vi "GlobalUI.vi"() -> ()   [LabVIEW 2012]
uses:
  typedefs/Scan Parameters.ctl
  typedefs/HWsettings.ctl
  typedefs/Stage Parameters.ctl
  typedefs/ScanMode.ctl
  classes/MCCPMT.lvclass
  typedefs/Scan Type.ctl
  typedefs/Move Type.ctl
  typedefs/MicroscopeEvent.ctl
  typedefs/Filenaming.ctl
panel:
  in  "Reading threshold defaults":dbl[](array[numeric])=[0.0, 0.0, 0.0]
  in  "Reading thresholds":dbl[](array[numeric])=[0.0, 0.0, 0.0]
  in  "Filenaming Mode":T1
  out "Microscope Events":refnum<queue>
  in  "configuration file":path=path "C:/Users/Trent/Dropbox/Shared/Jeremy/microscoper 2012/ConfigFiles/Jeremy.ini"
  out "SW Initializing":bool
  out "Image Initialized":bool
  out "Number of scans to average":u32=1
  in  "Stage":refnum<k7>(container)
  in  "Stage Serial Number":i32=94839332
  out "# elements in queue":i32
  out "Rotation Acquire Ready?":bool
  in  "Move Type":T2=enum."Continuous"
  in  "Scan Type":T3=enum."Point"
  out "Integration Time (ms)":u32=83
  in  "MakeAcquireButtonFalse":bool
  out "acquiring":bool
  out "MCCPMT":refnum<class "MCCPMT.lvclass">
  out "error out":errorcluster
  in  "detector startup delay (ms)":u32=1000
  out "Stage Position (mm)":dbl=77.27864837646484
  out "Samples Averaged":dbl=82.0
  out "Samples Per Line":dbl=6150.0
  out "Flyback samples":dbl=25.0
  in  "Zoom":dbl=4.0
  in  "Target position mm":dbl=82.4884 step=0.025 format="%_6g"
  in  "Target position mm 2":dbl=78.45775 step=0.025 format="%_6g"
  in  "Target position mm 3":dbl=77.0 step=0.025 format="%_6g"
  in  "Velocity mm/s":sgl=5.0 min=0.01 max=10 step=0.1
  out "PMT3 on":bool
  out "PMT2 on":bool
  out "PMT1 on":bool
  in  "Get Stage Position":bool
  in  "Acquire":bool
  out "Cursor Y (V)":dbl=-0.8695652173913044
  out "Cursor X (V)":dbl=1.2532299741602064
  out "Detector Timebase divisor":i32=13
  out "Actual write rate":dbl=18761.72607879925
  out "Expected write rate":dbl=18761.72607879925
  out "Actual read rate":dbl=1538461.5384615385
  out "must be an integer":dbl=82.0
  out "Galvo Timebase divisor":i32=1066
  out "Intensity x label":string="Time Elapsed (s)"
  in  "Save Path":path=path "C:/Users/Trent/Documents/Jeremy"
  out "Intensity vs Stage Position (mm)":cluster{dbl[], dbl[]}[](array[cluster])=[{[0.0, 1.3910799026489258, 1.5990915298461914, 1.8071036338806152, 2.015115261077881, 2.2071261405944824, 2.4151382446289062, 2.62214994430542, 2.8301620483398438, 3.0221729278564453, 3.230185031890869, 3.4381966590881348, 3.6462087631225586, 3.83821964263916, 4.046231746673584, 4.253243446350098, 4.4612555503845215, 4.653266429901123, 4.861278057098389, 5.0692901611328125, 5.277301788330078, 5.469313144683838, 5.6773247718811035, 5.884336948394775, 6.092348575592041, 6.284359455108643, 6.492371559143066, 6.700383186340332, 6.908395290374756, 7.100406169891357, 7.308418273925781], [0.000122149923780488, 0.00012203887195121974, 0.00012211684451219482, 0.00012205836509146326, 0.00012210857469512214, 0.00012208849085365822, 0.0001219922065548779, 0.0001221192073170731, 0.00012216291920731678, 0.00012211270960365853, 0.00012210562118902425, 0.00012214874237804877, 0.00012212511432926825, 0.00012211625381097538, 0.00012212097942073178, 0.00012209912347560983, 0.00012205127667682942, 0.00012203414634146332, 0.00012206781631097554, 0.00012200815548780514, 0.00012220367759146314, 0.00012232418064024334, 0.00012240865091463348, 0.0001225149771341453, 0.0001225834984756086, 0.00012261126143292585, 0.00012276897865853544, 0.00012285640243902307, 0.0001228445884146327, 0.00012293732850609658]}, {[0.0, 1.3910799026489258, 1.5990915298461914, 1.8071036338806152, 2.015115261077881, 2.2071261405944824, 2.4151382446289062, 2.62214994430542, 2.8301620483398438, 3.0221729278564453, 3.230185031890869, 3.4381966590881348, 3.6462087631225586, 3.83821964263916, 4.046231746673584, 4.253243446350098, 4.4612555503845215, 4.653266429901123, 4.861278057098389, 5.0692901611328125, 5.277301788330078, 5.469313144683838, 5.6773247718811035, 5.884336948394775, 6.092348575592041, 6.284359455108643, 6.492371559143066, 6.700383186340332, 6.908395290374756, 7.100406169891357, 7.308418273925781], [0.00013135659298780475, 0.00013157338033536578, 0.00013012616234756093, 0.00013111440548780457, 0.00013301646341463397, 0.0001317883955792678, 0.000130992721036585, 0.0001326821265243906, 0.0001315072217987802, 0.0001293440739329267, 0.00013089761814024363, 0.00013007063643292666, 0.00012964237804878018, 0.00013161945503048738, 0.00012965419207317062, 0.00012840544969512196, 0.00012788208841463418, 0.00012783955792682928, 0.00012841371951219504, 0.00012860569740853655, 0.00012810419207317093, 0.00012816326219512175, 0.00012866535823170694, 0.00012888568978658576, 0.0001280764291158539, 0.00012789980945121965, 0.0001284456173780486, 0.00013150131478658524, 0.00012812073170731704, 0.00012772318978658532]}, {[0.0, 1.3910799026489258, 1.5990915298461914, 1.8071036338806152, 2.015115261077881, 2.2071261405944824, 2.4151382446289062, 2.62214994430542, 2.8301620483398438, 3.0221729278564453, 3.230185031890869, 3.4381966590881348, 3.6462087631225586, 3.83821964263916, 4.046231746673584, 4.253243446350098, 4.4612555503845215, 4.653266429901123, 4.861278057098389, 5.0692901611328125, 5.277301788330078, 5.469313144683838, 5.6773247718811035, 5.884336948394775, 6.092348575592041, 6.284359455108643, 6.492371559143066, 6.700383186340332, 6.908395290374756, 7.100406169891357, 7.308418273925781], [0.0015331301638719503, 0.0015423486471036582, 0.0015469194931402445, 0.0015383738185975615, 0.001518318330792681, 0.0015139979420731706, 0.0015096173018292658, 0.00150134630335366, 0.0014566284489329268, 0.0014108739138719547, 0.0014768062118902425, 0.0014940812690548806, 0.0015152945312499973, 0.0015447988757621935, 0.0014241475609756108, 0.0014025462080792695, 0.0013903263719512208, 0.001438070388719513, 0.0014299364329268304, 0.0014168329077743902, 0.0014394319550304904, 0.001461583841463416, 0.0014690036394817024, 0.0014612311928353645, 0.0014412194169207292, 0.0014495364900914622, 0.001426015948932925, 0.0014652012957317051, 0.0014510108803353662, 0.0014339579268292664]}]
  out "Image intensities":dbl[](array[numeric])
  out "Images":dbl[][][](array[numeric])
  in  "Maximum frame diff":i32=1
  in  "Use Image Controls Min Max values for tiff":bool=TRUE
  in  "Autosave":bool
  in  "show flyback data":bool
  in  "disable averaging":bool
  in  "Sample Description":string="AXN static 25d"
  in  "Stokes Power (mW)":string="200"
  in  "Pump Power (mW)":string="5"
  in  "PMT3":dbl(slide)=0.7 min=0.0 max=1.0 step=0.01 scale=0.0..1.0
  in  "PMT2":dbl(slide)=0.7 min=0.0 max=1.0 step=0.01 scale=0.0..1.0
  in  "PMT1":dbl(slide)=0.6 min=0.0 max=1.0 step=0.01 scale=0.0..1.0 scale format="%#_1g"
  out "Grabbed all required frames? (image processor)":bool
  out "image  maximums":dbl[](array[numeric])=[250.0, 250.0, 500.0]
  out "image  minimums":dbl[](array[numeric])=[0.0, 0.0, 283.1435785060976]
  in  "status":string[](array[string])=["Initializing", "Setting parameters", "Initializing", "Setting parameters", "Initializing", "Setting parameters", "closing image data", "Setting acquire button to false", "Setting acquire button to false", "closing image data", "stopping acquisition", "Acquire sequence set", "closing image data", "post acquire", "acquiring", "initializing image data", "closing image data", "pre-acquiring", "initializing galvos and detectors", "preparing stage", "initializing image data", "closing image data", "Setting parameters", "Acquire sequence set", "Initializing", "Setting parameters", "Setting parameters", "Setting parameters", "initializing image data", "closing image data", "post acquire", "acquiring", "pre-acquiring", "initializing galvos and detectors", "preparing stage", "Setting parameters", "preparing to acquire", "Wait for event", "Setting acquire button to false", "stopping acquisition", "preparing to acquire", "Wait for event", "post acquire", "initializing image data", "acquiring", "Wait for event", "pre-acquiring", "initializing galvos and detectors", "enabling acquire buttons", "Setting parameters", "post acquire", "initializing image data", "acquiring", "pre-acquiring", "initializing galvos and detectors", "enabling acquire buttons", "Setting parameters", "Wait for event", "post acquire", "initializing image data", "acquiring", "pre-acquiring", "initializing galvos and detectors", "enabling acquire buttons", "Setting parameters", "Wait for event", "post acquire", "initializing image data", "acquiring", "Wait for event", "pre-acquiring", "initializing galvos and detectors", "enabling acquire buttons", "Setting parameters", "post acquire", "initializing image data", "acquiring", "Wait for event", "pre-acquiring", "initializing galvos and detectors", "enabling acquire buttons", "Setting parameters", "post acquire", "initializing image data", "acquiring", "pre-acquiring", "initializing galvos and detectors", "enabling acquire buttons", "Setting parameters", "Wait for event", "post acquire", "initializing image data", "acquiring", "pre-acquiring", "initializing galvos and detectors", "enabling acquire buttons", "Setting parameters", "Wait for event", "post acquire", "initializing image data", "acquiring", "Wait for event", "pre-acquiring", "initializing galvos and detectors", "enabling acquire buttons", "Setting parameters", "post acquire", "initializing image data", "acquiring", "Wait for event", "pre-acquiring", "initializing galvos and detectors", "enabling acquire buttons", "Setting parameters", "Wait for event", "Wait for event", "post acquire", "initializing image data", "acquiring", "pre-acquiring", "initializing galvos and detectors", "enabling acquire buttons", "Setting parameters", "Wait for event", "post acquire", "initializing image data", "acquiring", "pre-acquiring", "initializing galvos and detectors", "preparing stage", "Setting parameters", "preparing to acquire", "Wait for event", "moving stage to 3rd option", "Setting parameters", "Initializing", "Setting parameters", "Initializing", "Setting parameters", "Bumming", "restoring to default state", "Bumming", "stopping acquisition", "Bumming", "preparing to acquire", "closing image data", "post acquire", "processing image", "initializing image data", "processing image", "initializing image data", "acquiring", "pre-acquiring", "initializing galvos and detectors", "preparing stage", "getting parameters", "preparing to acquire", "Bumming", "moving stage to 3rd option", "getting parameters", "Bumming", "stopping acquisition", "restoring to default state", "post acquire", "processing image", "initializing image data", "processing image", "initializing image data", "closing image data", "acquiring", "pre-acquiring", "initializing galvos and detectors", "preparing stage", "getting parameters", "preparing to acquire", "Bumming", "restoring to default state", "Bumming", "stopping acquisition", "Bumming", "preparing to acquire", "post acquire", "processing image", "initializing image data", "processing image", "initializing image data", "acquiring", "pre-acquiring", "initializing galvos and detectors", "preparing stage", "getting parameters", "preparing to acquire", "Bumming", "moving stage to 3rd option", "getting parameters", "Bumming", "stopping acquisition", "restoring to default state", "post acquire", "processing image", "initializing image data", "processing image", "initializing image data", "closing image data", "acquiring", "pre-acquiring", "initializing galvos and detectors", "preparing stage", "getting parameters", "preparing to acquire", "Bumming", "restoring to default state", "Bumming", "stopping acquisition", "Bumming", "preparing to acquire", "post acquire", "processing image", "initializing image data", "processing image", "initializing image data", "acquiring", "pre-acquiring", "initializing galvos and detectors", "preparing stage", "getting parameters", "preparing to acquire", "Bumming", "moving stage to 3rd option", "getting parameters", "Bumming", "stopping acquisition", "restoring to default state", "post acquire", "processing image", "initializing image data", "processing image", "initializing image data", "acquiring", "pre-acquiring", "initializing galvos and detectors", "preparing stage", "getting parameters", "preparing to acquire", "Bumming", "restoring to default state", "Bumming", "stopping acquisition", "Bumming", "preparing to acquire", "closing image data", "post acquire", "reinitializing image data parameters", "closing image data", "acquiring", "pre-acquiring", "initializing galvos and detectors", "enabling acquire buttons", "getting parameters", "moving stage to 3rd option", "getting parameters", "Bumming", "post acquire", "processing image", "initializing image data", "processing image", "initializing image data", "acquiring", "pre-acquiring", "initializing galvos and detectors", "preparing stage", "getting parameters", "preparing to acquire", "Bumming", "stopping acquisition", "restoring to default state", "post acquire", "processing image", "initializing image data", "processing image", "initializing image data", "acquiring", "pre-acquiring", "initializing galvos and detectors", "preparing stage", "getting parameters", "preparing to acquire", "Bumming", "restoring to default state", "Bumming", "stopping acquisition", "Bumming", "preparing to acquire", "closing image data", "post acquire", "processing image", "initializing image data", "acquiring", "pre-acquiring", "initializing galvos and detectors", "preparing stage", "getting parameters", "preparing to acquire", "Bumming", "restoring to default state", "Bumming", "stopping acquisition", "Bumming", "preparing to acquire", "closing image data", "post acquire", "processing image", "initializing image data", "processing image", "initializing image data", "processing image", "initializing image data", "acquiring", "pre-acquiring", "initializing galvos and detectors", "preparing stage", "getting parameters", "preparing to acquire", "Bumming", "getting parameters", "Bumming", "restoring to default state", "Bumming", "stopping acquisition", "Bumming", "preparing to acquire", "closing image data", "post acquire", "processing image", "initializing image data", "closing image data", "acquiring", "pre-acquiring", "initializing galvos and detectors", "enabling acquire buttons", "getting parameters", "Bumming", "post acquire", "processing image", "initializing image data", "closing image data", "acquiring", "pre-acquiring", "initializing galvos and detectors", "preparing stage", "getting parameters", "preparing to acquire", "Bumming", "restoring to default state", "Bumming", "stopping acquisition", "Bumming", "preparing to acquire", "post acquire", "processing image", "initializing image data", "processing image", "initializing image data", "acquiring", "pre-acquiring", "initializing galvos and detectors", "preparing stage", "getting parameters", "preparing to acquire", "Bumming", "moving stage to 3rd option", "getting parameters", "Bumming", "restoring to default state", "Bumming", "stopping acquisition", "Bumming", "stopping acquisition", "restoring to default state", "preparing to acquire", "post acquire", "processing image", "initializing image data", "processing image", "initializing image data", "acquiring", "pre-acquiring", "initializing galvos and detectors", "preparing stage", "getting parameters", "preparing to acquire", "Bumming", "restoring to default state", "Bumming", "stopping acquisition", "Bumming", "preparing to acquire", "closing image data", "post acquire", "reinitializing image data parameters", "acquiring", "pre-acquiring", "initializing galvos and detectors", "enabling acquire buttons", "getting parameters", "Bumming", "closing image data", "post acquire", "reinitializing image data parameters", "acquiring", "pre-acquiring", "initializing galvos and detectors", "enabling acquire buttons", "getting parameters", "Bumming", "closing image data", "post acquire", "reinitializing image data parameters", "closing image data", "acquiring", "pre-acquiring", "initializing galvos and detectors", "enabling acquire buttons", "getting parameters", "Bumming", "post acquire", "processing image", "initializing image data", "closing image data", "acquiring", "pre-acquiring", "initializing galvos and detectors", "enabling acquire buttons", "getting parameters", "Bumming", "post acquire", "reinitializing image data parameters", "acquiring", "pre-acquiring", "initializing galvos and detectors", "enabling acquire buttons", "getting parameters", "moving stage to 3rd option", "getting parameters", "Bumming", "closing image data", "post acquire", "processing image", "initializing image data", "closing image data", "acquiring", "pre-acquiring", "initializing galvos and detectors", "enabling acquire buttons", "getting parameters", "Bumming", "post acquire", "reinitializing image data parameters", "acquiring", "pre-acquiring", "initializing galvos and detectors", "enabling acquire buttons", "getting parameters", "moving stage to 3rd option", "getting parameters", "Bumming", "closing image data", "post acquire", "reinitializing image data parameters", "acquiring", "pre-acquiring", "initializing galvos and detectors", "enabling acquire buttons", "getting parameters", "moving stage to 3rd option", "getting parameters", "Bumming", "closing image data", "post acquire", "processing image", "initializing image data", "acquiring", "pre-acquiring", "initializing galvos and detectors", "preparing stage", "getting parameters", "preparing to acquire", "Bumming", "restoring to default state", "Bumming", "stopping acquisition", "Bumming", "preparing to acquire", "closing image data", "post acquire", "reinitializing image data parameters", "closing image data", "acquiring", "pre-acquiring", "initializing galvos and detectors", "enabling acquire buttons", "getting parameters", "moving stage to 3rd option", "getting parameters", "Bumming", "post acquire", "reinitializing image data parameters", "acquiring", "pre-acquiring", "initializing galvos and detectors", "enabling acquire buttons", "getting parameters", "moving stage to 3rd option", "getting parameters", "Bumming", "closing image data", "post acquire", "reinitializing image data parameters", "acquiring", "pre-acquiring", "initializing galvos and detectors", "enabling acquire buttons", "getting parameters", "moving stage to 3rd option", "getting parameters", "Bumming", "closing image data", "post acquire", "reinitializing image data parameters", "acquiring", "pre-acquiring", "initializing galvos and detectors", "enabling acquire buttons", "getting parameters", "moving stage to 3rd option", "getting parameters", "Bumming", "closing image data", "post acquire", "reinitializing image data parameters", "acquiring", "pre-acquiring", "initializing galvos and detectors", "enabling acquire buttons", "getting parameters", "moving stage to 3rd option", "getting parameters", "Bumming", "Bumming", "closing image data", "post acquire", "processing image", "initializing image data", "acquiring", "pre-acquiring", "initializing galvos and detectors", "preparing stage", "getting parameters", "preparing to acquire", "Bumming", "restoring to default state", "Bumming", "stopping acquisition", "Bumming", "preparing to acquire", "closing image data", "post acquire", "reinitializing image data parameters", "acquiring", "pre-acquiring", "initializing galvos and detectors", "enabling acquire buttons", "getting parameters", "moving stage to 3rd option", "getting parameters", "Bumming", "closing image data", "post acquire", "reinitializing image data parameters", "closing image data", "acquiring", "pre-acquiring", "initializing galvos and detectors", "enabling acquire buttons", "getting parameters", "moving stage to 3rd option", "getting parameters", "Bumming", "post acquire", "reinitializing image data parameters", "closing image data", "acquiring", "pre-acquiring", "initializing galvos and detectors", "enabling acquire buttons", "getting parameters", "moving stage to 3rd option", "getting parameters", "Bumming", "post acquire", "reinitializing image data parameters", "acquiring", "pre-acquiring", "initializing galvos and detectors", "enabling acquire buttons", "getting parameters", "moving stage to 3rd option", "getting parameters", "Bumming", "closing image data", "post acquire", "processing image", "initializing image data", "closing image data", "acquiring", "pre-acquiring", "initializing galvos and detectors", "preparing stage", "getting parameters", "preparing to acquire", "Bumming", "restoring to default state", "Bumming", "stopping acquisition", "Bumming", "preparing to acquire", "Bumming", "Bumming", "Bumming", "post acquire", "reinitializing image data parameters", "acquiring", "pre-acquiring", "initializing galvos and detectors", "enabling acquire buttons", "getting parameters", "moving stage to 2nd option", "getting parameters", "Bumming", "closing image data", "post acquire", "reinitializing image data parameters", "acquiring", "pre-acquiring", "initializing galvos and detectors", "enabling acquire buttons", "getting parameters", "moving stage to 1st option", "getting parameters", "Bumming", "closing image data", "post acquire", "processing image", "initializing image data", "closing image data", "acquiring", "pre-acquiring", "initializing galvos and detectors", "enabling acquire buttons", "getting parameters", "Bumming", "post acquire", "processing image", "initializing image data", "acquiring", "pre-acquiring", "initializing galvos and detectors", "enabling acquire buttons", "getting parameters", "Bumming", "closing image data", "post acquire", "processing image", "initializing image data", "acquiring", "pre-acquiring", "initializing galvos and detectors", "enabling acquire buttons", "getting parameters", "Bumming", "closing image data", "post acquire", "reinitializing image data parameters", "acquiring", "pre-acquiring", "initializing galvos and detectors", "enabling acquire buttons", "getting parameters", "moving stage to 3rd option", "getting parameters", "Bumming", "closing image data", "post acquire", "reinitializing image data parameters", "acquiring", "pre-acquiring", "initializing galvos and detectors", "enabling acquire buttons", "getting parameters", "moving stage to 3rd option", "getting parameters", "Bumming", "closing image data", "post acquire", "reinitializing image data parameters", "acquiring", "pre-acquiring", "initializing galvos and detectors", "enabling acquire buttons", "getting parameters", "moving stage to 3rd option", "getting parameters", "Bumming", "closing image data", "post acquire", "reinitializing image data parameters", "acquiring", "pre-acquiring", "initializing galvos and detectors", "enabling acquire buttons", "getting parameters", "moving stage to 3rd option", "getting parameters", "Bumming", "closing image data", "post acquire", "processing image", "initializing image data", "acquiring", "pre-acquiring", "initializing galvos and detectors", "preparing stage", "getting parameters", "preparing to acquire", "Bumming", "restoring to default state", "Bumming", "stopping acquisition", "Bumming", "preparing to acquire", "closing image data", "post acquire", "processing image", "initializing image data", "acquiring", "pre-acquiring", "initializing galvos and detectors", "enabling acquire buttons", "getting parameters", "Bumming", "closing image data", "post acquire", "processing image", "initializing image data", "acquiring", "pre-acquiring", "initializing galvos and detectors", "enabling acquire buttons", "getting parameters", "Bumming", "closing image data", "post acquire", "processing image", "initializing image data", "acquiring", "pre-acquiring", "initializing galvos and detectors", "enabling acquire buttons", "getting parameters", "Bumming", "closing image data", "post acquire", "processing image", "initializing image data", "acquiring", "pre-acquiring", "initializing galvos and detectors", "enabling acquire buttons", "getting parameters", "Bumming", "closing image data", "post acquire", "processing image", "initializing image data", "acquiring", "pre-acquiring", "initializing galvos and detectors", "preparing stage", "getting parameters", "preparing to acquire", "Bumming", "restoring to default state", "Bumming", "stopping acquisition", "Bumming", "preparing to acquire", "closing image data", "post acquire", "processing image", "initializing image data", "acquiring", "pre-acquiring", "initializing galvos and detectors", "preparing stage", "getting parameters", "preparing to acquire", "Bumming", "restoring to default state", "Bumming", "stopping acquisition", "Bumming", "preparing to acquire", "closing image data", "post acquire", "processing image", "initializing image data", "processing image", "initializing image data", "acquiring", "pre-acquiring", "initializing galvos and detectors", "preparing stage", "getting parameters", "preparing to acquire", "Bumming", "Bumming", "moving stage to 3rd option", "getting parameters", "Bumming", "Bumming", "Bumming", "Bumming", "Bumming", "Bumming", "Bumming", "Bumming", "Bumming", "Bumming", "stopping acquisition", "restoring to default state", "post acquire", "processing image", "initializing image data", "processing image", "initializing image data", "acquiring", "pre-acquiring", "initializing galvos and detectors", "preparing stage", "getting parameters", "preparing to acquire", "Bumming", "restoring to default state", "Bumming", "stopping acquisition", "Bumming", "stopping acquisition", "restoring to default state", "preparing to acquire", "post acquire", "processing image", "initializing image data", "processing image", "initializing image data", "acquiring", "pre-acquiring", "initializing galvos and detectors", "preparing stage", "getting parameters", "preparing to acquire", "Bumming", "restoring to default state", "Bumming", "stopping acquisition", "Bumming", "preparing to acquire", "closing image data", "post acquire", "processing image", "initializing image data", "acquiring", "pre-acquiring", "initializing galvos and detectors", "preparing stage", "getting parameters", "preparing to acquire", "Bumming", "Bumming", "Getting ready for you", "getting parameters", "starting up!"]
  in  "Stage Acquire Parameters":T4={"Scan Mode"=enum."None", "Start position mm"=79.5, "End position mm"=83.0, "Velocity um/sec (continuous)"=100.0, "Step size microns (discrete)"=100.0, "Frames to grab (grab)"=1} {"Frames to grab (grab)" min=1 step=1; "Velocity um/sec (continuous)" min=0.1 max=10000.0 step=1.0 format="%.1f"; "End position mm" min=0.0 max=220.0 step=0.1 format="%_6g"; "Start position mm" min=0.0 max=220.0 step=0.1 format="%_6g"; "Step size microns (discrete)" min=0.1 max=1000.0 step=1.0 format="%.1f"}
  in  "Hardware Settings":T6={"Galvo Channels"="Dev1/ao0:1", "Detector Channels"="Dev1/ai0:2", "Galvo Trigger"="/Dev1/ai/StartTrigger", "Shutter Lines"=["Dev1/port0/line7"], "Max Acquisition Rate"=5000000.0, "Recommended Acquisition Rate"=5000000.0, "Galvo Write Rate"=2500000.0, "Max Timebase Frequency (Hz)"=20000000.0, "MCC Shutter Lines"=["Dev0/AuxPort/Do1", "Dev0/AuxPort/Do2"], "Detector Task"="", "Shutter Tasks"=[], "Galvo Task"="", "Digital Image Multiplier"=[100.0, 100.0, 100.0]} {"Max Acquisition Rate" min=0.0 max=5000000.0 step=100000.0}
  in  "Scan Parameters":T7={"x pixels"=50, "x voltage min"=-7.0, "x voltage max"=9.0, "y voltage min"=-8.75, "y voltage max"=7.25, "fill frac"=0.5, "Zoom"=4.0, "BiDi"=FALSE, "scan rate (ms/line)"=4.0} {"fill frac" min=0.0 step=0.05 format="%.2f"; "y voltage max" format="%0.2p"; "y voltage min" format="%.2f"; "x voltage max" format="%0.2p"; "x voltage min" format="%0.2p"}
  out "Images Displayed":i32
  out "Images Acquired":i32
  # "Stage Variables"
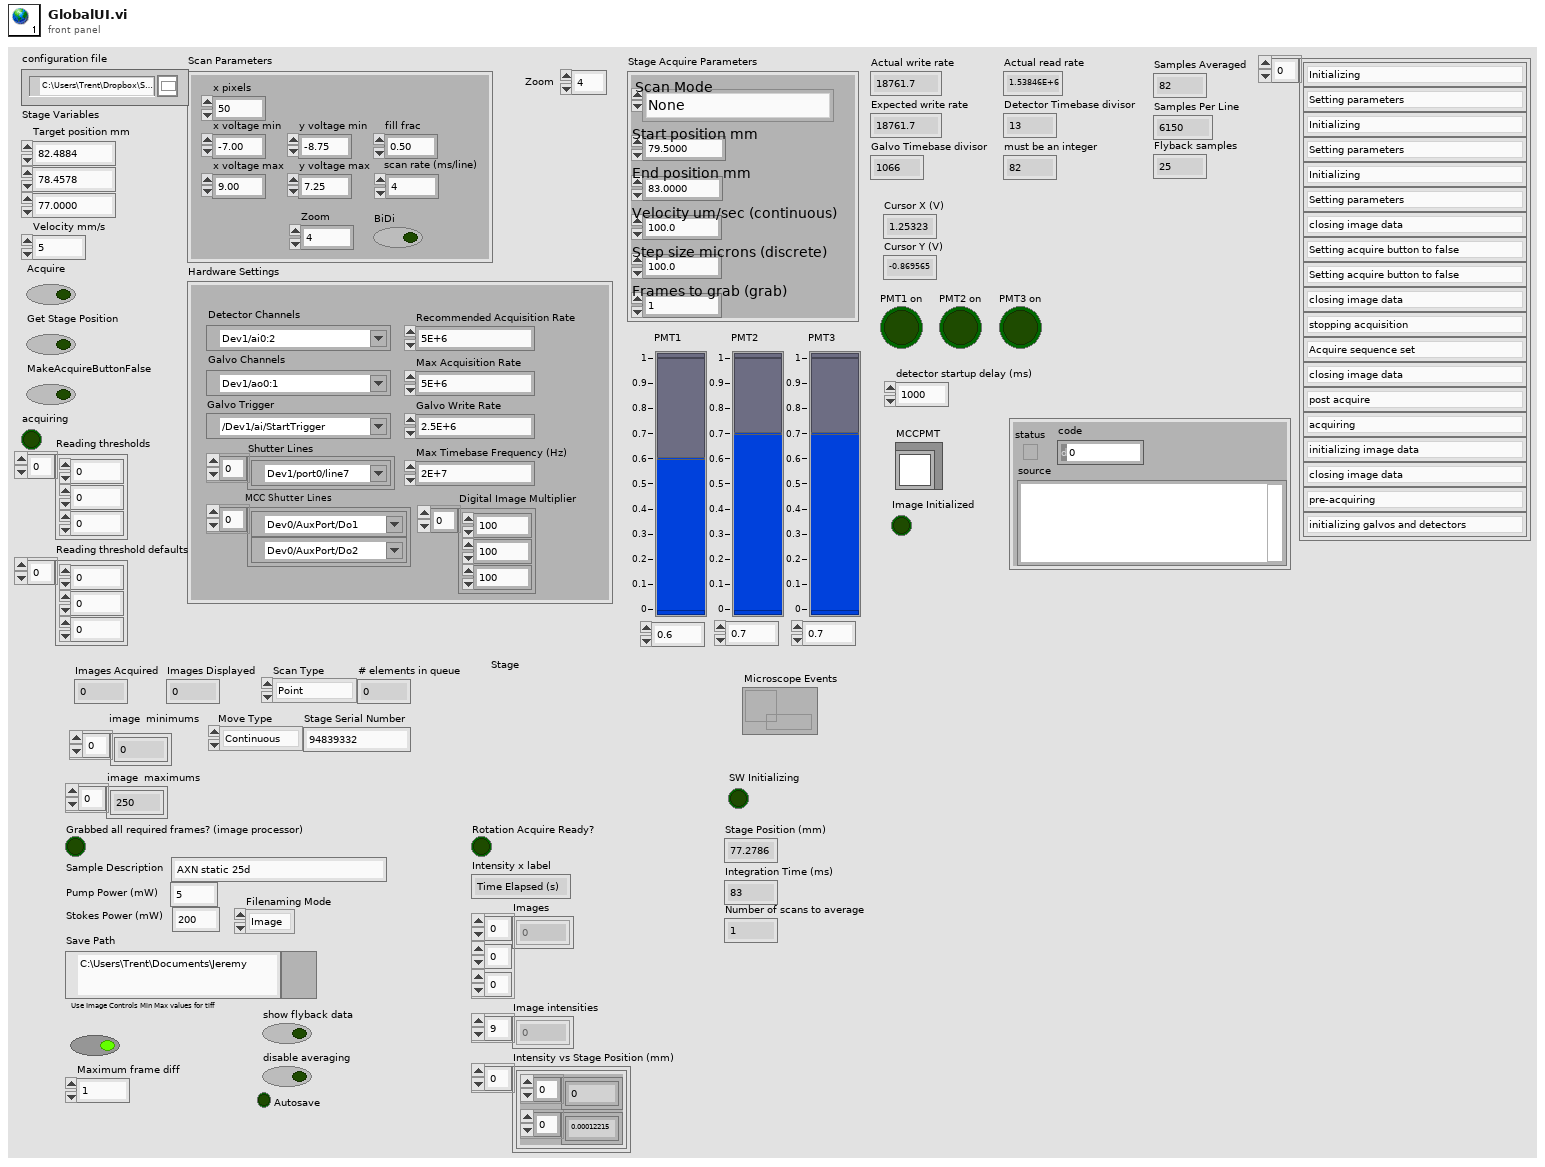
[diagram p1: front panel]
types:
  T1 = typedef "Filenaming.ctl" = enum16{"Image", "Just Description"}
  T2 = typedef "Move Type.ctl" = enum16{"None", "Continuous", "Discrete"}
  T3 = typedef "Scan Type.ctl" = enum16{"None", "Point", "Full Image Continuous", "Full Image Grab"}
  T4 = typedef "Stage Parameters.ctl" = cluster{"Scan Mode":T5, "Start position mm":dbl, "End position mm":dbl, "Velocity um/sec (continuous)":dbl, "Step size microns (discrete)":dbl, "Frames to grab (grab)":i32}
  T5 = typedef "ScanMode.ctl" = enum16{"None", "Continuous", "Point Scan (CH3 cursor)", "Point Scan Move (CH3 cursor)", "Grab", "Grab Move Stage", "Grab Move Z-stage", "Cont. Move Z-stage", "Spec Move Stage", "Spec Move Cont", "Surf Calib"}
  T6 = typedef "HWsettings.ctl" = cluster{"Galvo Channels":tag, "Detector Channels":tag, "Galvo Trigger":tag, "Shutter Lines":tag[], "Max Acquisition Rate":dbl, "Recommended Acquisition Rate":dbl, "Galvo Write Rate":dbl, "Max Timebase Frequency (Hz)":dbl, "MCC Shutter Lines":refnum<k21>[], "Detector Task":refnum<k21>, "Shutter Tasks":refnum<k21>[], "Galvo Task":refnum<k21>, "Digital Image Multiplier":dbl[]}
  T7 = typedef "Scan Parameters.ctl" = cluster{"x pixels":i32, "x voltage min":dbl, "x voltage max":dbl, "y voltage min":dbl, "y voltage max":dbl, "fill frac":dbl, "Zoom":dbl, "BiDi":bool, "scan rate (ms/line)":dbl}
diagram:
